vi "Synchronize Control Panel.vi"(8 "error in (no error)":errorcluster, 11 "Cryomagnetics Power Supply in":refnum<class "Cryomagnetics Power Supply.lvclass">) -> (0 "error out":errorcluster, 3 "Cryomagnetics Power Supply out":refnum<class "Cryomagnetics Power Supply.lvclass">)   [LabVIEW 2015, in "Cryomagnetics Power Supply.lvclass"]
uses:
  Cryomagnetics Power Supply.lvclass
  Cryomagnetics Control Panel Data.ctl
  Sweep mode.ctl
  Instrument/Read VISA Resource.vi
  Instrument/Write VISA Resource.vi
  OO Devices/Device/Device.lvclass
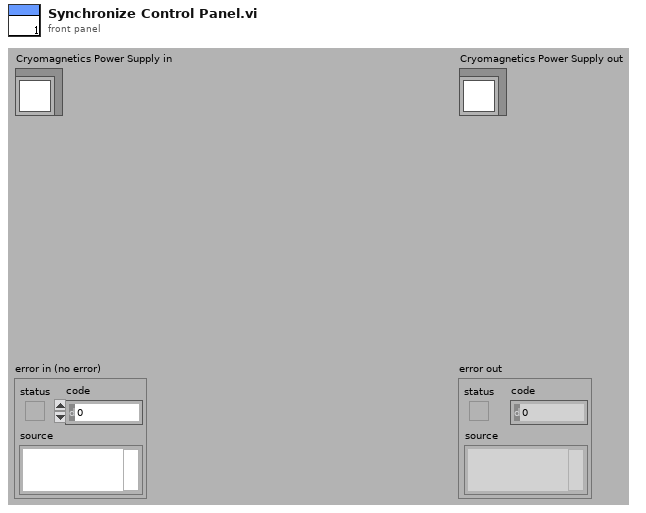
[diagram p1: front panel]
types:
  T1 = typedef "Cryomagnetics Control Panel Data.ctl" = cluster{"Persistent switch heater":bool, "Rates, A/s":dbl[], "Ranges, A":dbl[], "High limit, kG":dbl, "Low limit, kG":dbl, "Sweep ":T2, "Fast rate":dbl}
  T2 = typedef "Sweep mode.ctl" = cluster{"zero":bool, "sweep up":bool, "sweep down":bool, "fast sweep":bool}
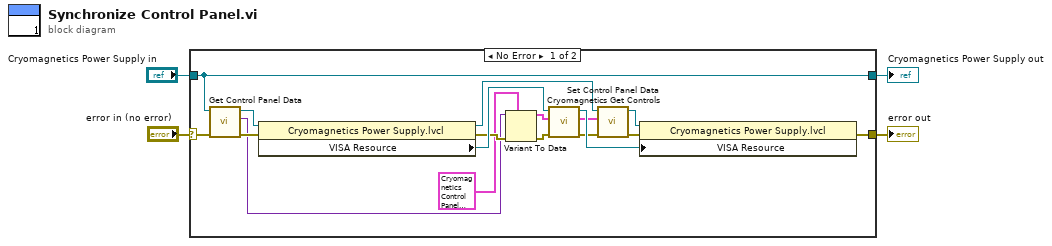
[diagram p0: block diagram]
diagram:
  n1 = case shown="No Error" "error in (no error)" {
    selector: "error in (no error)" -> [w8 w23]
    tunnel: [w7 w23] -> w3
    tunnel: [w9 w22] -> w1
    tunnel: "Cryomagnetics Power Supply in" -> [w9 w22]
    frame No Error {
      n2 = call-dynamic "Get Control Panel Data.vi"("error in (no error)"=w8, "Device in"=w9) -> ("error out"=w15:errorcluster, "Data"=w13:variant, "Device out"=w10:refnum<class "Cryomagnetics Power Supply.lvclass">)  [unwired: 7 in]
      n3 = property class="Cryomagnetics Power Supply.lvcl"(reference=w10, error in=w15) -> (reference out=w17:refnum<class "Cryomagnetics Power Supply.lvclass">, error out=w16:errorcluster, "VISA Resource"=w21:refnum<visa-resource-name>)
      n4 = Variant To Data(error in=w16, type=T1 {"Persistent switch heater"=FALSE, "Rates, A/s"=[0.01, 0.05, 0.0001, 0.0001, 0.0001], "Ranges, A"=[50.0, 76.9, 80.0, 85.0, 100.0], "High limit, kG"=0.01, "Low limit, kG"=0.0, "Sweep "={"zero"=FALSE, "sweep up"=FALSE, "sweep down"=FALSE, "fast sweep"=FALSE}, "Fast rate"=0.0} ("Data"), Variant=w13) -> (data=w6:T1, error out=w12:errorcluster)
      n5 = call "Cryomagnetics Get Controls.vi"("error in (no error)"=w12, "Data in"=w6, "VISA resource name"=w21) -> ("error out"=w14:errorcluster, "Data out"=w5:T1, "VISA Resource Name Out"=w20:refnum<visa-resource-name>)  [unwired: 6 in]
      n6 = call "Set Control Panel Data.vi"("error in (no error)"=w14, "Data"=w5, "Device in"=w17) -> ("error out"=w19:errorcluster, "Device out"=w18:refnum<class "Cryomagnetics Power Supply.lvclass">)  [unwired: 7 in]
      n7 = property class="Cryomagnetics Power Supply.lvcl"(reference=w18, error in=w19, "VISA Resource"=w20) -> (error out=w7:errorcluster)  [unwired: 1 out]
    }
    frame Error {
    }
  }
  "error out" <- w3
  "Cryomagnetics Power Supply out" <- w1
